vi "R_set2Set_Point.vi"(0 "range":i8(ring) items=["no range", "2 Ohms", "20 Ohms", "200 Ohms", "2 kOhms", "20 kOhms", "200 kOhms", "2 MOhms"], 1 "Widerstand_Target":dbl) -> (3 "SetPoint":dbl)   [LabVIEW 2010]
panel:
  out "Ohm/SetPoint":dbl
  out "Range":dbl
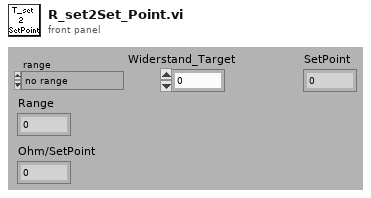
[diagram p1: front panel]
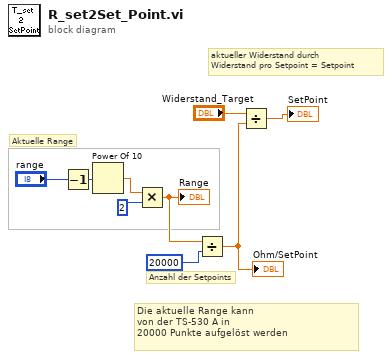
[diagram p0: block diagram]
diagram:
  # "aktueller Widerstand durch\nWiderstand pro Setpoint = Setpoint"
  # "Die aktuelle Range kann\nvon der TS-530 A in\n20000 Punkte aufgelöst werden"
  # "Anzahl der Setpoints"
  # "Aktuelle Range"
  n1 = Decrement(x="range") -> (x-1=w7:i8)
  n2 = Power Of 10(x=w7) -> (10^x=w9:dbl)
  n3 = Multiply(x=w9, y=2) -> (x*y=w5:dbl)
  "Range" <- w5
  n4 = Divide(x=w5, y=20000) -> (x/y=w2:dbl)
  "Ohm/SetPoint" <- w2
  n5 = Divide(x="Widerstand_Target", y=w2) -> (x/y=→"SetPoint":dbl)
